vi "LN2 Dewar Spuelen.vi"(6 "Aktionen":T1, 10 "LN2 Spülen?":bool) -> (2 "LN2 Spülen?":bool)   [LabVIEW 2020, in "Erweiterte Konfig.lvlib"]
uses:
  Erweiterte Konfig.lvlib
  Aktionen LN2 Dewar Spuelen.ctl
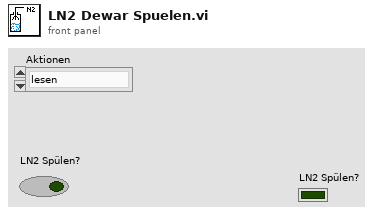
[diagram p1: front panel]
types:
  T1 = typedef "Erweiterte Konfig.lvlib/Aktionen LN2 Dewar Spuelen.ctl" = enum16{"lesen", "schreiben", "prüfen"}
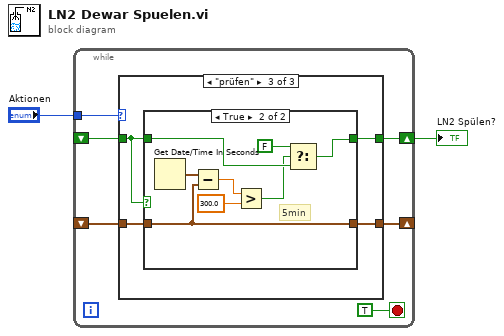
[diagram p0: block diagram]
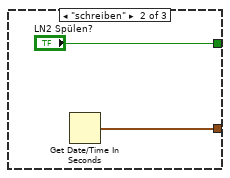
[diagram p3: hidden frame]
diagram:
  n1 = while {
    tunnel: "Aktionen" -> [w7]
    shift-right: [w6] -> w1
    shift-left: _ -> [w3]
    shift-right: [w5] -> _
    shift-left: _ -> [w4]
    stop <- TRUE stop-if-true
    n2 = case shown="\"prüfen\"" w7 {
      tunnel: [w10 "LN2 Spülen?" w14] -> w6
      tunnel: [w9 w11 w13] -> w5
      tunnel: w4 -> [w9 _ w16]
      tunnel: w3 -> [w10 _ w15]
      frame "lesen", Default {
      }
      frame "schreiben" {
        n3 = Get Date/Time In Seconds() -> (seconds since 1Jan1904=w11:timestamp)
      }
      frame "prüfen" {
        n4 = case shown="True" w15 {
          tunnel: w16 -> [w17 w19]
          tunnel: w15 -> [w18 w23]
          tunnel: [w18 w20] -> w14
          tunnel: [w17 w19] -> w13
          frame False {
          }
          frame True {
            # "5min"
            n5 = Get Date/Time In Seconds() -> (seconds since 1Jan1904=w26:timestamp)
            n6 = Subtract(x=w26, y=w19) -> (x-y=w24:dbl)
            n7 = Greater?(x=w24, y=300.0) -> (0:w22:bool)
            n8 = Select(t=FALSE, s=w22, f=w23) -> (s? t:f=w20:bool)
          }
        }
      }
    }
  }
  "LN2 Spülen?" <- w1
